vi "Create All Message Queues.vi"(8 "error in (no error)":errorcluster) -> (0 "error out":errorcluster, 3 "Message Queues out":T1)   [LabVIEW 2018, in "Message Queue.lvlib"]
doc: "This VI creates and initializes all the message queues for your application. If your application requires more than one message queue, right-click the \"Message Queues\" constant above and select Open Type Def. Add the new Message Queue(s) to the type definition, then initialize them in this VI."
uses:
  Message Queue.lvlib
  All Message Queues.ctl
  Message Cluster.ctl
  Enqueue Message (Single).vi
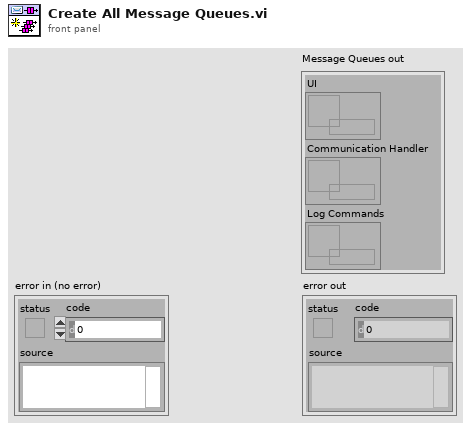
[diagram p1: front panel]
types:
  T1 = typedef "Message Queue.lvlib/All Message Queues.ctl" = cluster{"UI":refnum<queue>, "Communication Handler":refnum<queue>, "Log Commands":refnum<queue>}
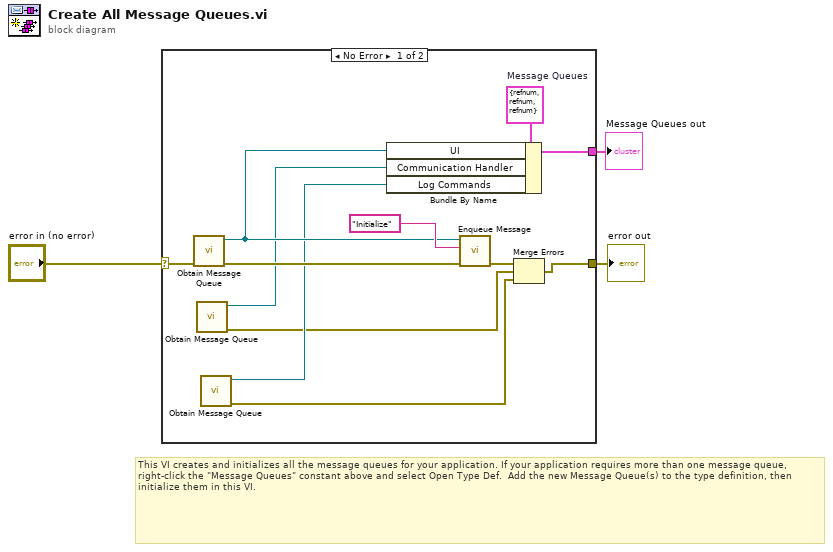
[diagram p0: block diagram]
diagram:
  # "This VI creates and initializes all the message queues for your application. If your application requires more than one message queue, right-click the \"Message Queues\" constant above and select Open Type Def.  Add the new Message Queue(s) to the type definition, then initialize them in this VI."
  n1 = case shown="No Error" "error in (no error)" {
    selector: "error in (no error)" -> [w13 w16]
    tunnel: [w5 w16] -> w3
    tunnel: [w14 _] -> w2
    frame No Error {
      w15 = T1 {"UI"=refnum, "Communication Handler"=refnum, "Log Commands"=refnum}  # Message Queues
      n2 = call "Obtain Message Queue.vi"("error in (no error)"=w13) -> ("error out"=w12:errorcluster, "Message Queue"=w10:refnum<queue>)  [unwired: 9 in]
      n3 = call "Obtain Message Queue.vi"() -> ("error out"=w6:errorcluster, "Message Queue"=w9:refnum<queue>)  [unwired: 10 in]
      n4 = call "Obtain Message Queue.vi"() -> ("error out"=w4:errorcluster, "Message Queue"=w8:refnum<queue>)  [unwired: 10 in]
      n5 = Bundle By Name(cluster=w15, "UI"=w10, "Communication Handler"=w9, "Log Commands"=w8) -> (w14:T1)
      n6 = call-poly "Enqueue Message.vi"("error in (no error)"=w12, "Message"="Initialize", "Message Queue"=w10) -> ("error out"=w7:errorcluster)  [unwired: 7 in, 1 out]
      n7 = Merge Errors(w7, w6, w4) -> (w5:errorcluster)
    }
    frame Error {
    }
  }
  "Message Queues out" <- w2
  "error out" <- w3
